vi "Main_06a.vi"() -> ()   [LabVIEW 2023]
uses:
  <vilib>/Utility/error.llb/Trim Whitespace One-Sided.vi
panel:
  out "Answer":i64
  out "Array 2":i64[](array[numeric])
  out "Array":i32[](array[numeric])
  out "number Array":i64[][](array[numeric])
  in  "Puzzle":string="Time:        41     66     72     66\nDistance:   244   1047   1228   1040"
  in  "Example":string="Time:      7  15   30\nDistance:  9  40  200"
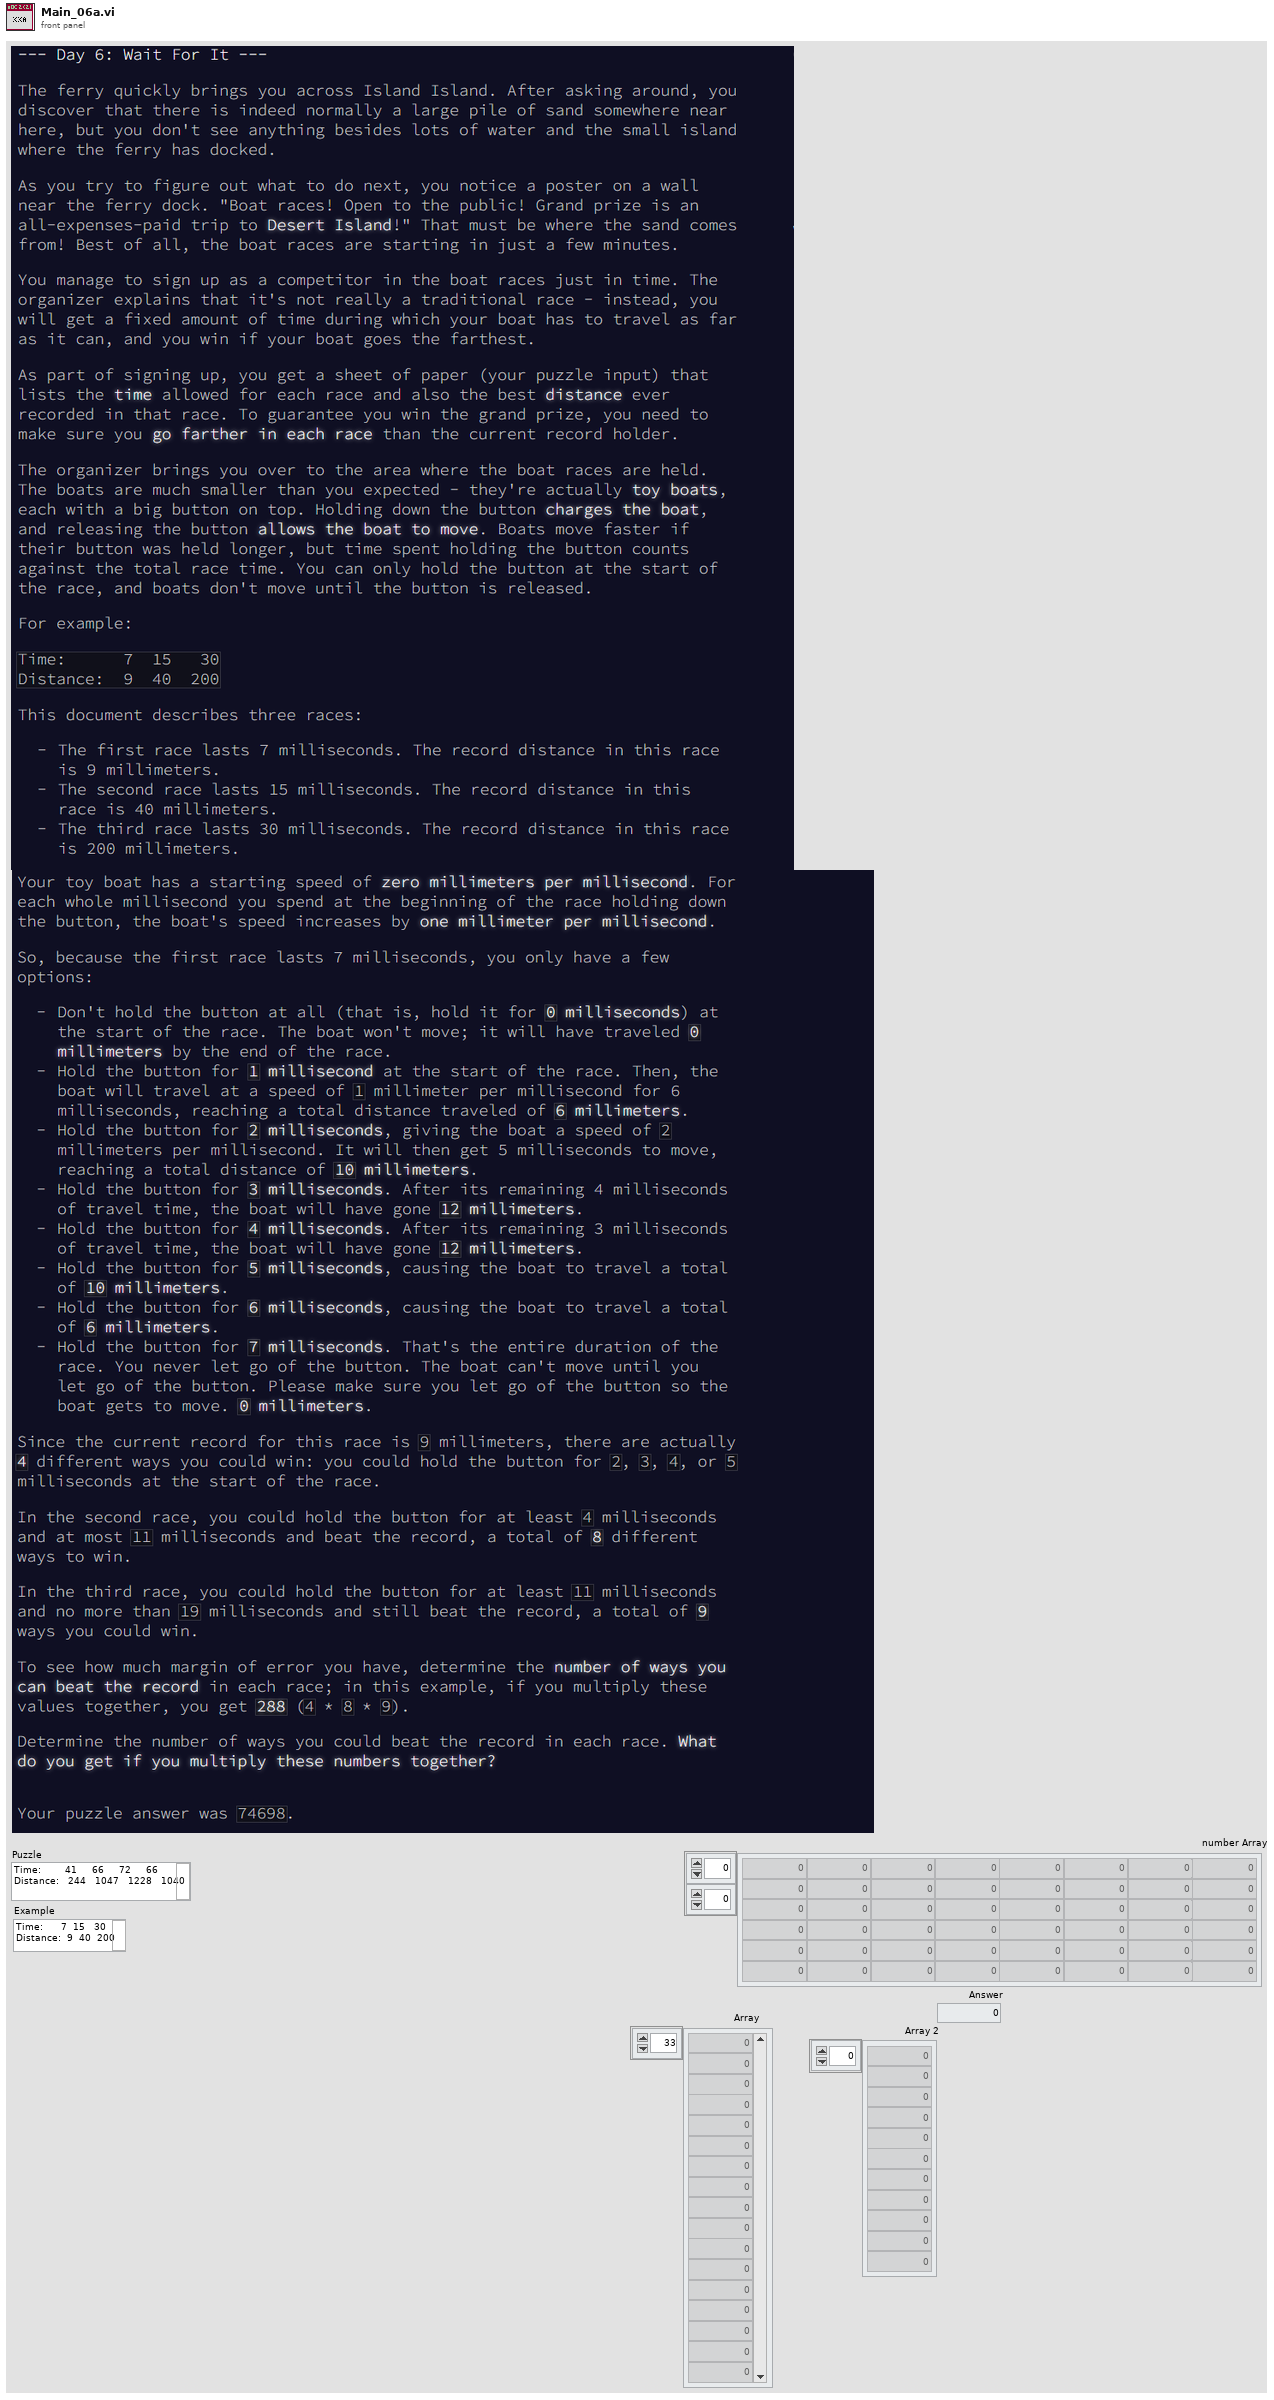
[diagram p1: front panel]
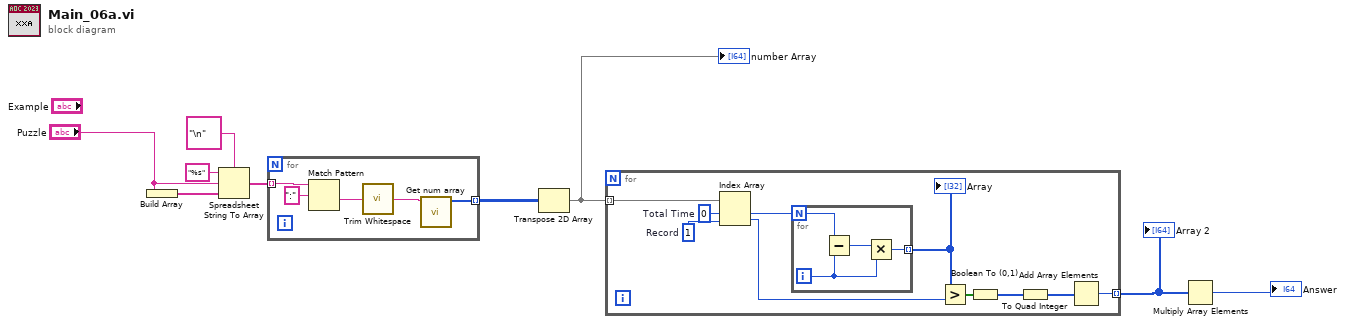
[diagram p0: block diagram]
diagram:
  n1 = Build Array("Puzzle") -> (w9:string[])
  n2 = Spreadsheet String To Array(delimiter (Tab)="\n", format string="%s", spreadsheet string="Puzzle", array type (2D Dbl)=w9) -> (array=w6:string[])
  n3 = for {
    tunnel: w6 -> [w14] mode=indexing
    tunnel: [w10] -> w5 mode=indexing
    n4 = Match Pattern(string=w14, regular expression=":") -> (after substring=w12:string)  [unwired: 1 in, 3 out]
    n5 = call <vilib>:"Trim Whitespace.vi"("string"=w12) -> ("trimmed string"=w11:string)  [unwired: 1 in]
    n6 = call "Get num array.vi"("number String"=w11) -> ("number Array"=w10:i64[])  [unwired: 10 in]
  }
  n7 = Transpose 2D Array(2D array=w5) -> (transposed array=w4:i64[][])
  "number Array" <- w4
  n8 = for {
    tunnel: w4 -> [w24] mode=indexing
    tunnel: [w16] -> w2 mode=indexing
    w22 = 1  # Record
    w23 = 0  # Total Time
    n9 = Index Array(array=w24, index #1=w23, index #2=w22) -> (element #1=w21:i64, element #2=w19:i64)
    n10 = for {
      N: w21 -> [w28]
      tunnel: [w25] -> w20 mode=indexing
      i -> [w26]
      n11 = Subtract(x=w28, y=w26) -> (x-y=w27:i32)
      n12 = Multiply(x=w27, y=w26) -> (x*y=w25:i32)
    }
    "Array" <- w20
    n13 = Greater?(x=w20, y=w19) -> (0:w18:bool[])
    n14 = Boolean To (0,1)(Boolean=w18) -> (0, 1=w17:i16[])
    n15 = To Quad Integer(1:w17) -> (0:w15:i64[])
    n16 = Add Array Elements(numeric array=w15) -> (sum=w16:i64)
  }
  "Array 2" <- w2
  n17 = Multiply Array Elements(1:w2) -> (0:→"Answer":i64)
